vi "Create JSON Schema (Interactive).vi"(8 "error in (no error)":errorcluster, 9 "LV Object":variant, 11 "JSON Schema in":string) -> (0 "error out":errorcluster, 3 "JSON Schema out":string)   [LabVIEW 2019, in "JSON-Schema.lvlib"]
doc: "Interactively generates a JSON Schema for <b>LV object</b>, add additional, user-defined metadata, and merges with any <b>JSON Schema in</b>."
uses:
  <vilib>/JDP Science/JSONtext/Next JSON Value.vi
  <vilib>/JDP Science/JSONtext/String Subset.vi
  <vilib>/JDP Science/JSONtext/Parsing/Advance past next JSON Value (inlined COPY).vi
  <vilib>/JDP Science/JSONtext/Parsing/Advance past whitespace.vi
  <vilib>/JDP Science/JSONtext/Parsing/Advance past String.vi
  <vilib>/JDP Science/JSONtext/Parsing/Advance past Number.vi
  <vilib>/JDP Science/JSONtext/Parsing/Advance past Line Ending.vi
  <vilib>/JDP Science/JSONtext/Parsing/Parse Full Path or Item Name.vi
  <vilib>/JDP Science/JSONtext/Parsing/Advance past Array.vi
  <vilib>/JDP Science/JSONtext/Parsing/Advance past Object.vi
  <vilib>/JDP Science/JSONtext/support/Error Cluster From Code.vi
  <vilib>/JDP Science/JSONtext/Offset/Find Item Locations by Path.vi
  JSON-Schema.lvlib
  <vilib>/JDP Science/JSONtext/JSONtext.lvlib
  <vilib>/Utility/Data Type/NI_Data Type.lvlib
panel:
  in  "Write":bool
  in  "Table":bool
  in  "Load":bool
  in  "Path":path
  in  "Description":string
  in  "Title":string
  in  "Table":string[][](table)
  # "- This program will take a LV object and convert to a JSON Schema.\n   - If you don't wire anything to the LV Object terminal you can Load Object by Path.\n- After the initial JSON Schema is created, the Table will be filled with the relevant information.\n- Please update as appropriate and click Add Table to Schema.\n- Note: running Load Object will clear the previously loaded object and table."
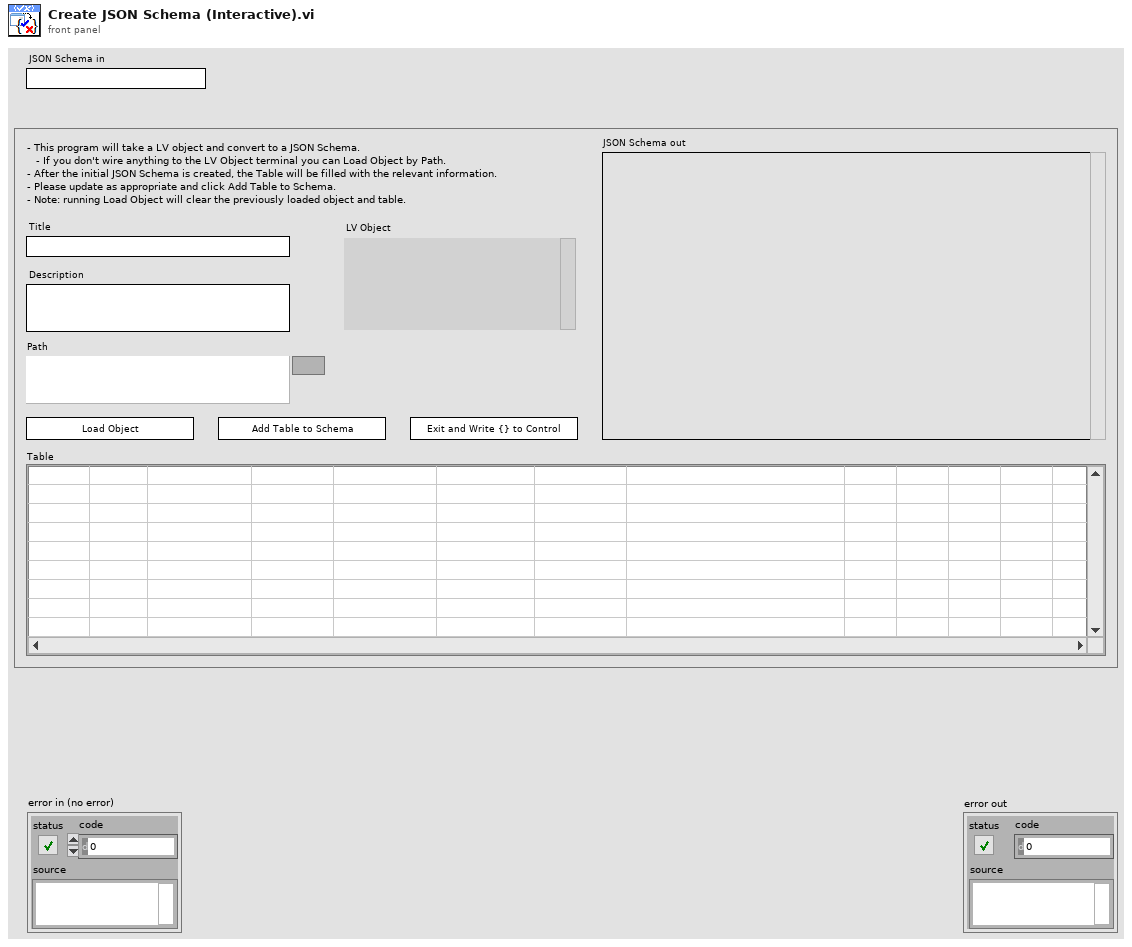
[diagram p1: front panel]
types:
  T1 = enum32{"Invalid", "Standard", "Closed", "Hidden", "Minimized", "Maximized"}
  T2 = enum32{"invalid app kind", "Development System", "Run Time System", "Student Edition", "Embedded LabVIEW", "Evaluation", "Custom"}
  T3 = cluster{"Core":cluster{"Current VI Reference":refnum<vi>, "Close Panel on Exit?":bool}, "JSON Schema":string, "LV Object":variant}
  T4 = cluster{"Current VI Reference":refnum<vi>, "Close Panel on Exit?":bool}
  T5 = typedef "JSONtext.lvlib/JSON Value Type.ctl" = enum16{"Not a JSON Value", "JSON Object", "JSON Array", "String", "Number", "true", "false", "null"}
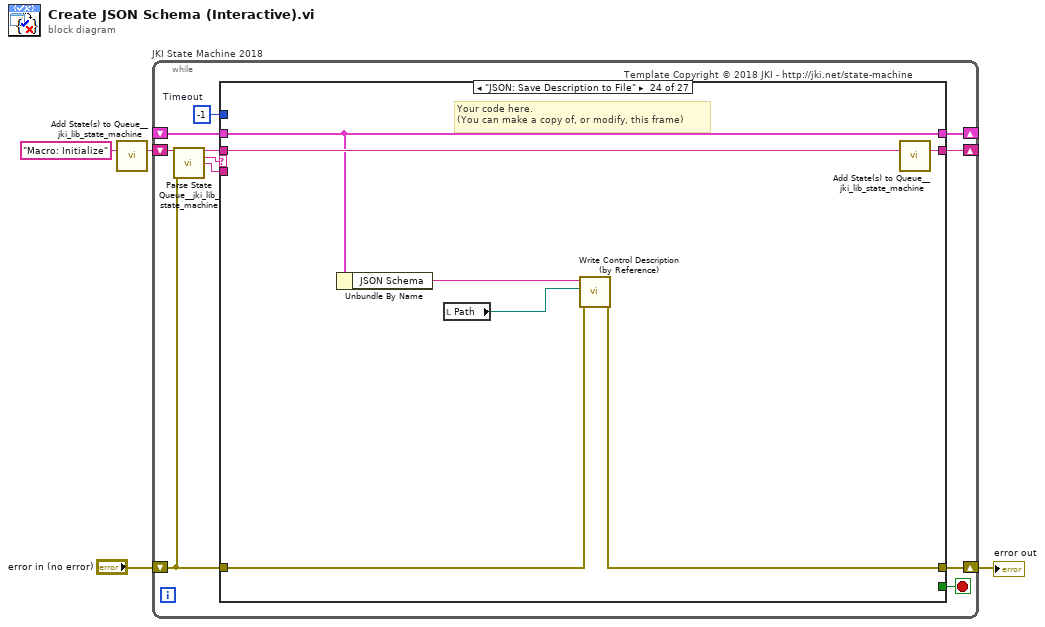
[diagram p0: block diagram]
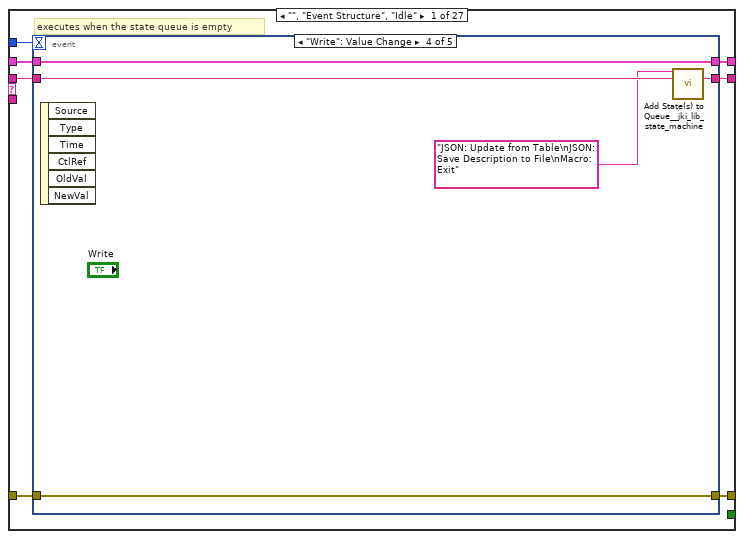
[diagram p2: hidden frame]
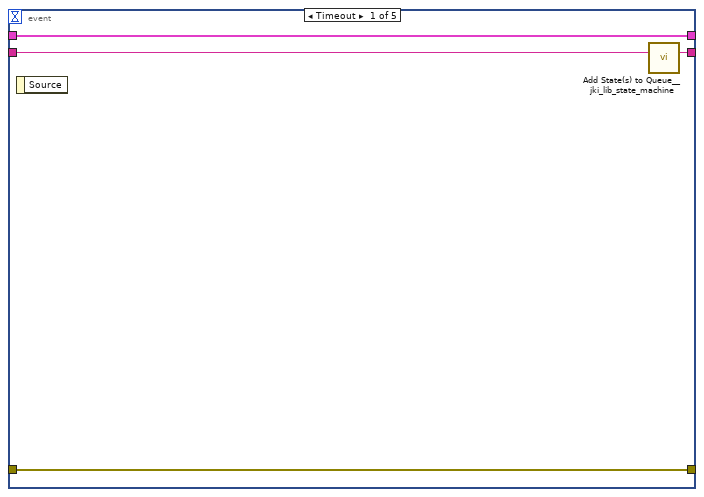
[diagram p3: hidden frame]
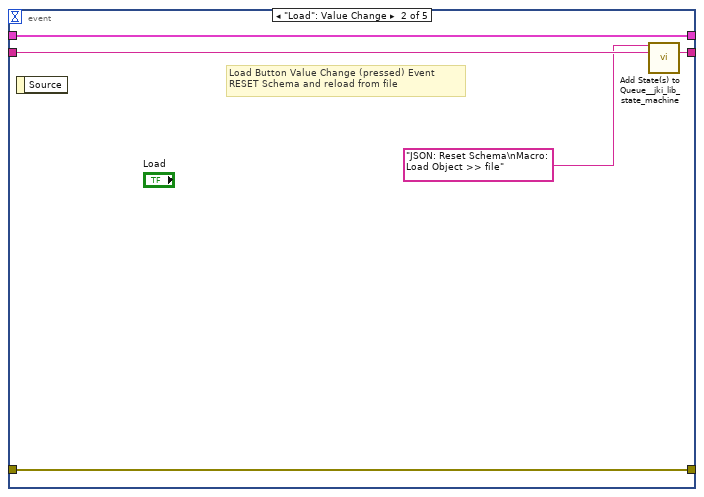
[diagram p4: hidden frame]
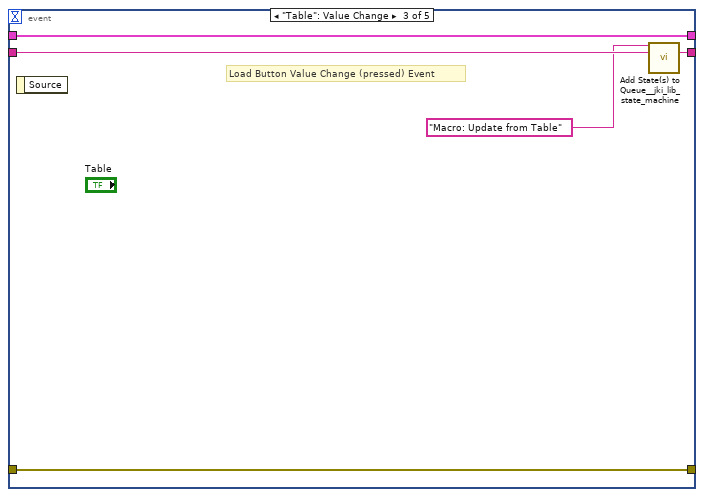
[diagram p5: hidden frame]
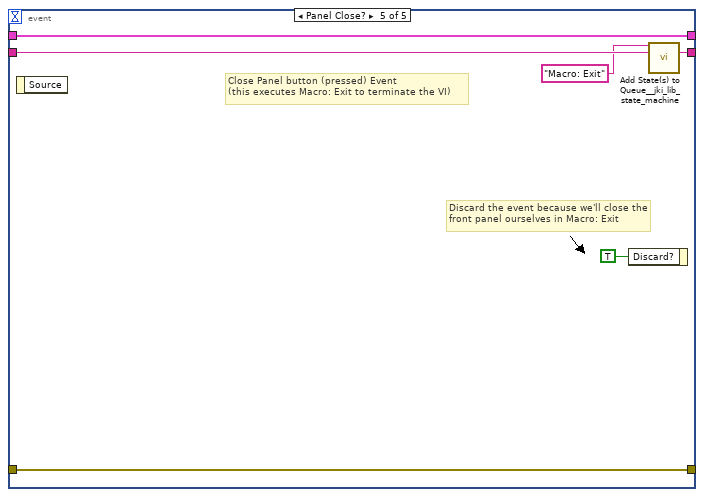
[diagram p6: hidden frame]
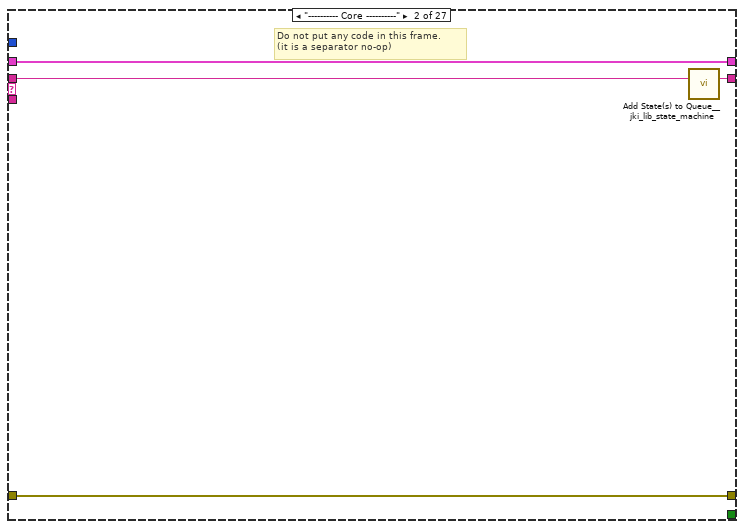
[diagram p7: hidden frame]
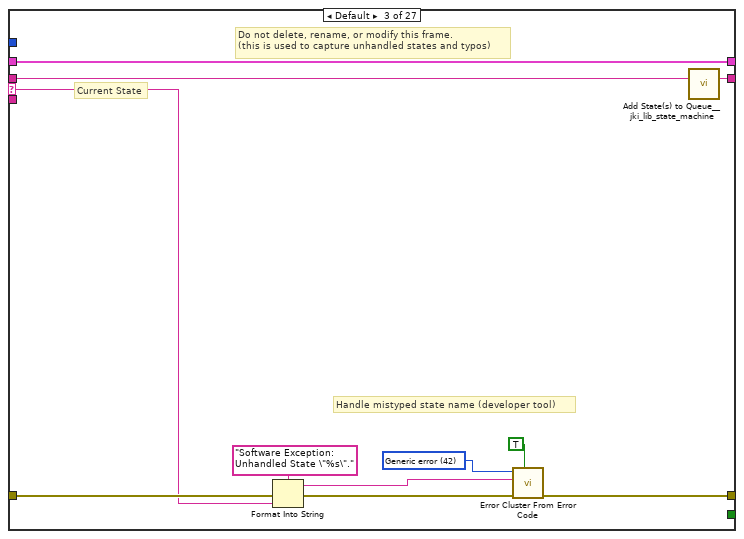
[diagram p8: hidden frame]
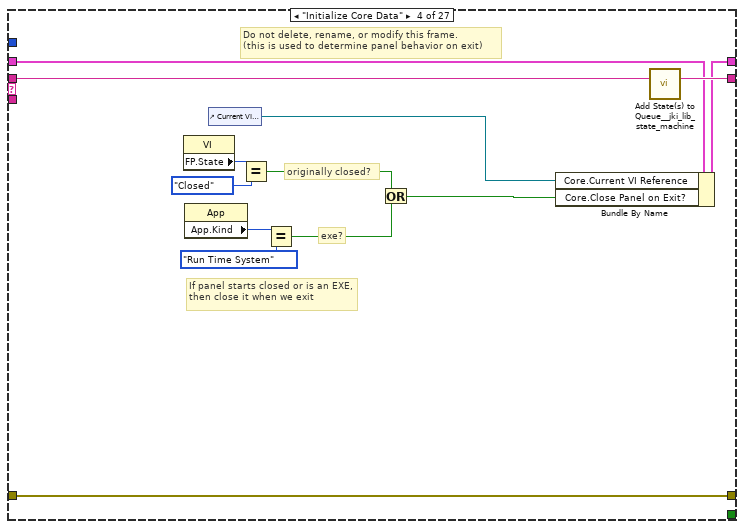
[diagram p9: hidden frame]
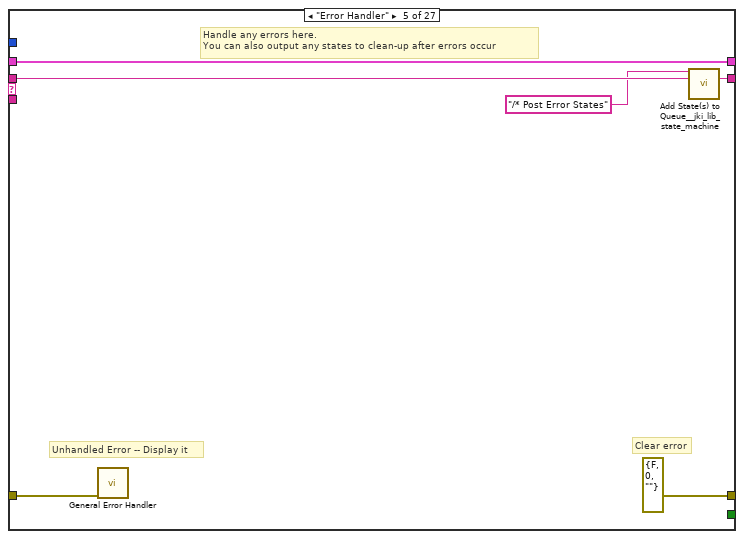
[diagram p10: hidden frame]
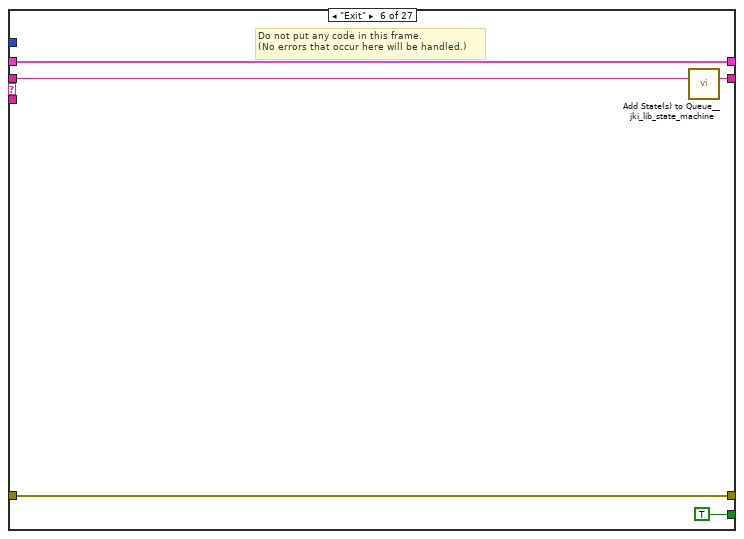
[diagram p11: hidden frame]
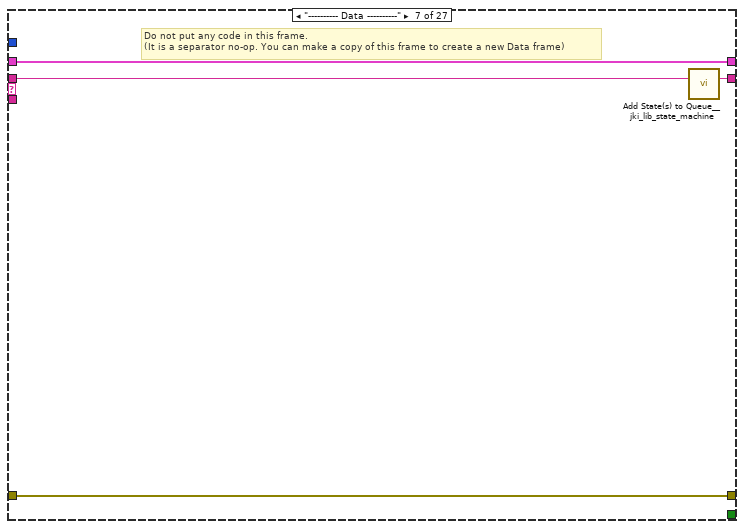
[diagram p12: hidden frame]
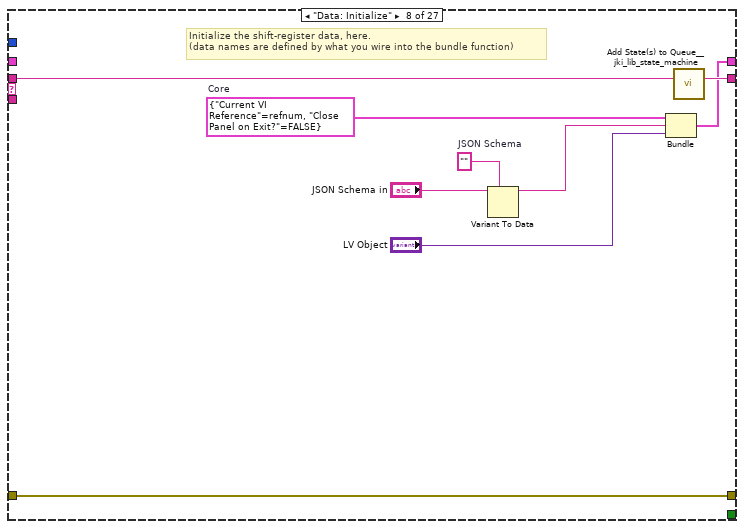
[diagram p13: hidden frame]
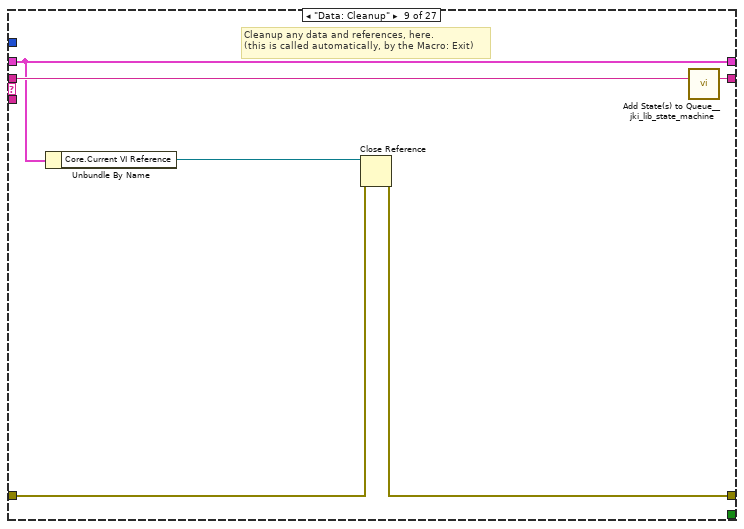
[diagram p14: hidden frame]
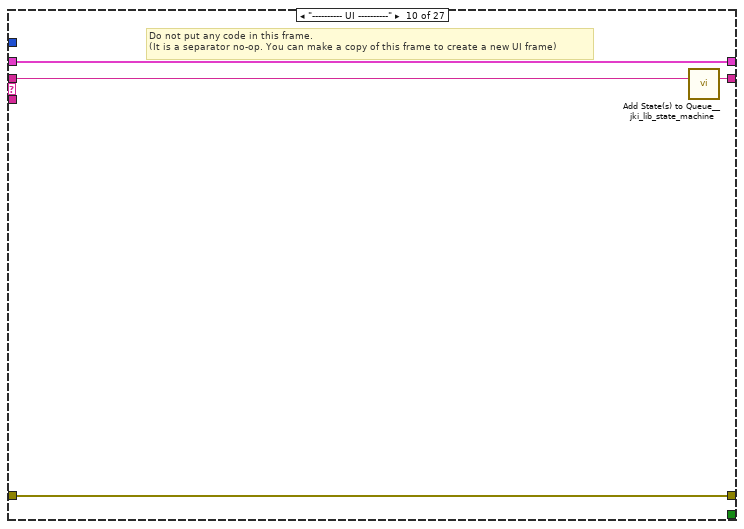
[diagram p15: hidden frame]
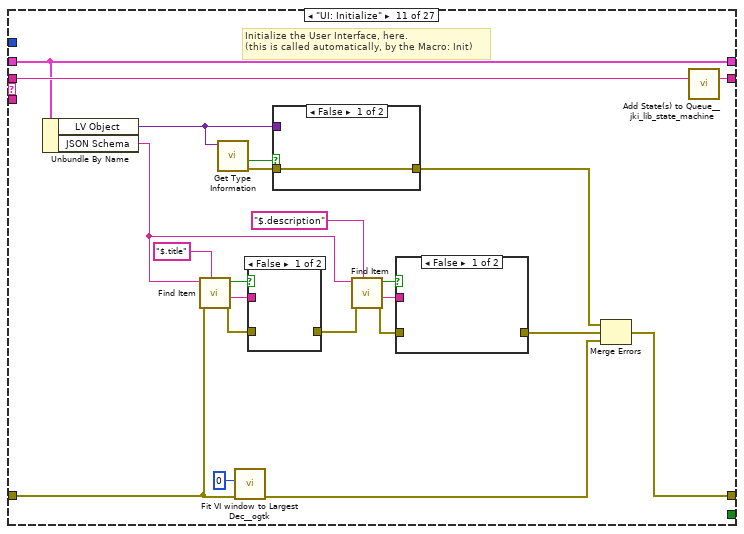
[diagram p16: hidden frame]
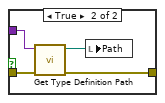
[diagram p17: hidden frame]
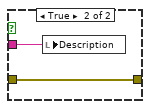
[diagram p18: hidden frame]
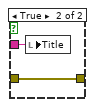
[diagram p19: hidden frame]
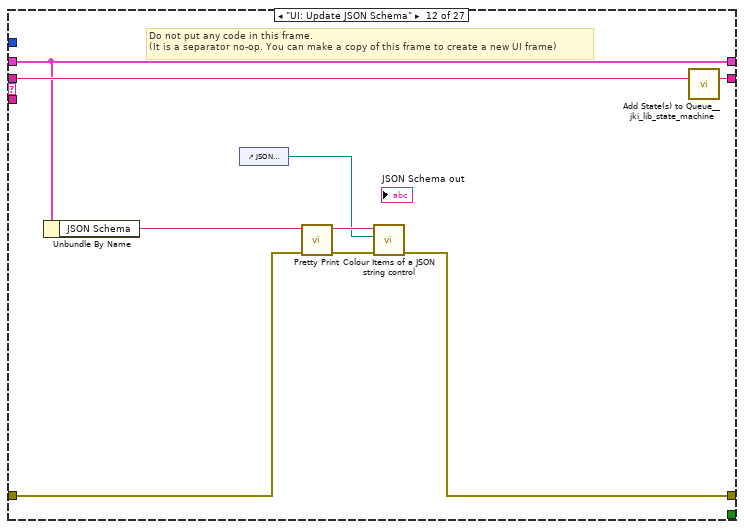
[diagram p20: hidden frame]
diagram:
  n1 = call <vilib>:"Add State(s) to Queue__jki_lib_state_machine.vi"("State(s) in (\"\")"="Macro: Initialize") -> ("States Out"=w4:string)  [unwired: 14 in]
  n2 = while "JKI State Machine 2018" {
    shift-right: [w8] -> _
    shift-left: _ -> [w7]
    shift-right: [w11] -> w1
    shift-left: "error in (no error)" -> [w5]
    shift-right: [w10] -> _
    shift-left: w4 -> [w12]
    stop <- w9 stop-if-true
    w6 = -1  # Timeout
    # "Template Copyright © 2018 JKI - http://jki.net/state-machine"
    n3 = call <vilib>:"Parse State Queue__jki_lib_state_machine.vi"("State Queue"=w12, "Error In (no error)"=w5) -> ("Remaining States"=w14:string, "Current State"=w15:string, "Arguments"=w13:string)  [unwired: 11 in]
    n4 = case shown="\"JSON: Save Description to File\"" w15 {
      selector: w15 -> [_ _ w52 _ _ _ _ _ _ _ _ _ _ _ _ _ _ _ _ _ _ _ _ _ _ _ _]
      tunnel: w14 -> [w22 w51 w56 w75 w81 w86 w90 w99 w105 w109 w131 w149 w155 w166 w235 w240 w252 w257 w267 w271 w281 w291 w303 w312 w321 w328 w337]
      tunnel: w13 -> [_ _ _ _ _ _ _ _ _ _ _ _ w150 w160 _ _ w248 _ _ _ _ _ _ _ _ _ _]
      tunnel: w7 -> [w20 w48 w54 w68 w78 w84 w87 _ w100 w106 w129 w146 w153 w162 w232 w237 w249 w254 w264 w268 w275 w285 w298 w308 w315 w325 w330]
      tunnel: [w19 w49 w58 w72 errorcluster {"status"=FALSE, "code"=0, "source"=""} ("error out") w83 w88 w94 w101 w107 w115 w142 w151 w163 w233 w238 w250 w255 w265 w269 w279 w289 w301 w310 w318 w323 w334] -> w11
      tunnel: w5 -> [w18 w49 w57 w72 w77 w83 w88 w94 w102 w107 w119 w141 w152 w164 w233 w238 w250 w255 w265 w269 w278 w288 w300 w309 w317 w322 w333]
      tunnel: [w21 w50 w55 w74 w80 w85 w89 w98 w104 w108 w130 w148 w154 w165 w234 w239 w251 w256 w266 w270 w280 w290 w302 w311 w320 w327 w336] -> w10
      tunnel: [_ _ _ _ _ TRUE _ _ _ _ _ _ _ _ _ _ _ _ _ _ _ _ _ _ _ _ _] -> w9
      tunnel: [w17 w48 w54 w73 w78 w84 w87 w97 w100 w106 w129 w146 w153 w162 w232 w237 w249 w254 w264 w268 w276 w286 w299 w308 w316 w325 w331] -> w8
      tunnel: w6 -> [w16 _ _ _ _ _ _ _ _ _ _ _ _ _ _ _ _ _ _ _ _ _ _ _ _ _ _]
      frame "", "Event Structure", "Idle" {
        # "executes when the state queue is empty"
        n5 = event shown="[3] \"Write\": Value Change" {
          selector: _ -> [_ _ _ _ _]
          dyn-events: _ -> [_ _ _ _ _]
          timeout: w16 -> [_ _ _ _ _]
          tunnel: w22 -> [w26 w31 w36 w41 w47]
          tunnel: [w25 w30 w35 w40 w46] -> w21
          tunnel: w20 -> [w23 w28 w33 w38 w44]
          tunnel: [w24 w29 w34 w39 w45] -> w19
          tunnel: w18 -> [w24 w29 w34 w39 w45]
          tunnel: [w23 w28 w33 w38 w44] -> w17
          event Timeout {
            n6 = event-data() -> ()  [unwired: 1 in, 1 out]
            n7 = call <vilib>:"Add State(s) to Queue__jki_lib_state_machine.vi"("State(s) in (\"\")"=w26) -> ("States Out"=w25:string)  [unwired: 14 in]
          }
          event "Load": Value Change {
            # "Load Button Value Change (pressed) Event\nRESET Schema and reload from file"
            n8 = event-data() -> ()  [unwired: 1 in, 1 out]
            n9 = call <vilib>:"Add State(s) to Queue__jki_lib_state_machine.vi"("State(s) in Front (\"\")"="JSON: Reset Schema\nMacro: Load Object >> file", "State(s) in (\"\")"=w31) -> ("States Out"=w30:string)  [unwired: 13 in]
          }
          event "Table": Value Change {
            # "Load Button Value Change (pressed) Event"
            n10 = event-data() -> ()  [unwired: 1 in, 1 out]
            n11 = call <vilib>:"Add State(s) to Queue__jki_lib_state_machine.vi"("State(s) in Front (\"\")"="Macro: Update from Table", "State(s) in (\"\")"=w36) -> ("States Out"=w35:string)  [unwired: 13 in]
          }
          event "Write": Value Change {
            n12 = event-data() -> ()  [unwired: 1 in, 6 out]
            n13 = call <vilib>:"Add State(s) to Queue__jki_lib_state_machine.vi"("State(s) in Front (\"\")"="JSON: Update from Table\nJSON: Save Description to File\nMacro: Exit", "State(s) in (\"\")"=w41) -> ("States Out"=w40:string)  [unwired: 13 in]
          }
          event Panel Close? {
            # "Discard the event because we'll close the front panel ourselves in Macro: Exit"
            # "Close Panel button (pressed) Event\n(this executes Macro: Exit to terminate the VI)"
            n14 = event-data() -> ()  [unwired: 1 in, 1 out]
            n15 = event-data("Discard?"=TRUE) -> ()  [unwired: 1 in, 1 out]
            n16 = call <vilib>:"Add State(s) to Queue__jki_lib_state_machine.vi"("State(s) in Front (\"\")"="Macro: Exit", "State(s) in (\"\")"=w47) -> ("States Out"=w46:string)  [unwired: 13 in]
          }
        }
      }
      frame "---------- Core ----------" {
        # "Do not put any code in this frame.\n(it is a separator no-op)"
        n17 = call <vilib>:"Add State(s) to Queue__jki_lib_state_machine.vi"("State(s) in (\"\")"=w51) -> ("States Out"=w50:string)  [unwired: 14 in]
      }
      frame Default {
        w61 = 42 items=["No error", "Argument error", "Memory is full", "Out of zone", "End of file", "File already open", "Generic file I/O error", "File not found", "File permission error", "Disk is full", "Duplicate path", "Too many files open", "System feature not enabled", "Resource file not found", "Cannot add resource", "Resource not found", "Image not found", "Image memory error", "Pen does not exist", "Config type invalid", "Config token not found", "Config parse error", "Config memory error", "Bad external code format", "Bad external code offset", "External code not present", "Null window", "Destroy window error", "Null menu", "Print aborted", "Bad print record", "Print driver error", "Windows error during printing", "Memory error during printing", "Print dialog error", "Generic print error", "Invalid device refnum", "Device not found", "Device parameter error", "Device unit error", "Cannot open device", "Device call aborted", "Generic error", "Cancelled by user", "Object ID too low", "Object ID too high", "Object not in heap", "Unknown heap", "Unknown object (invalid DefProc)", "Unknown object (DefProc not in table)", "Message out of range", "Invalid (null) method", "Unknown message", "Manager call not supported", "Bad address", "Network operation in progress", "Network operation timed out", "Connection is busy", "Network attribute not supported", "Network error", "Address in use", "System out of memory", "Connection aborted", "Connection refused", "Not connected", "Already connected", "Connection closed", "Initialization error (interapplication manager)", "Bad occurrence", "Wait on unbound occurrence handler", "Occurrence queue overflow", "Datalog type conflict", "Unused", "Unrecognized type (interapplication manager)", "Memory corrupt", "Failed to make temporary DLL", "Old CIN version", "Drag socket not found", "Failed to load drop-object", "Failed to register OLE object", "Failed to release OLE object", "Format specifier type mismatch", "Unknown format specifier", "Too few format specifiers", "Too many format specifiers", "Scan failed", "Newer CIN version", "Error converting to variant", "Runtime menu error", "Password tampered", "Variant attribute not found", "Incompatible variant data type", "Event data is not available", "Event Store is not present", "Occurrence is not found", "Event Queue is not created", "Event info is not available", "Refnum passed is NULL", "Error retrieving Class GUID", "Error retrieving CoClass GUID", "Error retrieving TypeLib GUID.", "Bad built application magic bytes.", "Specific driver is different from the specific driver associated with the Logical Name.", "There is no session opened to the class driver.", "Max Error", "MAX - Error with config objects", "MAX - Error loading configuration", "MAX - Group not supported"]
        # "Current State"
        # "Do not delete, rename, or modify this frame.\n(this is used to capture unhandled states and typos)"
        # "Handle mistyped state name (developer tool)"
        n18 = Format Into String(format string="Software Exception: Unhandled State \"%s\"." ("message"), error in=w57, w52) -> (resulting string=w60:string, error out=w59:errorcluster)  [unwired: 1 in]
        n19 = call <vilib>:"Error Cluster From Error Code.vi"("show call chain? (False)"=TRUE, "error in (no error)"=w59, "error message (\"\")"=w60, "error code (0)"=w61) -> ("error out"=w58:errorcluster)  [unwired: 5 in]
        n20 = call <vilib>:"Add State(s) to Queue__jki_lib_state_machine.vi"("State(s) in (\"\")"=w56) -> ("States Out"=w55:string)  [unwired: 14 in]
      }
      frame "Initialize Core Data" {
        # "Do not delete, rename, or modify this frame.\n(this is used to determine panel behavior on exit)"
        # "originally closed?"
        # "exe?"
        # "If panel starts closed or is an EXE, then close it when we exit"
        n21 = property class="VI"() -> ("FP.State"=w65:T1)  [unwired: 2 in, 2 out]
        n22 = property class="App"() -> ("App.Kind"=w71:T2)  [unwired: 2 in, 2 out]
        n23 = control-ref of="Current VI Reference"() -> (w66:refnum<vi>)
        n24 = Equal?(x=w65, y=T1."Closed" ("Front Panel Window:State")) -> (x = y?=w63:bool)
        n25 = Equal?(x=w71, y=T2."Run Time System" ("Application:Kind")) -> (x = y?=w69:bool)
        n26 = Or(x=w63, y=w69) -> (x .or. y?=w67:bool)
        n27 = Bundle By Name(cluster=w68, "Core.Current VI Reference"=w66, "Core.Close Panel on Exit?"=w67) -> (w73:T3)
        n28 = call <vilib>:"Add State(s) to Queue__jki_lib_state_machine.vi"("State(s) in (\"\")"=w75) -> ("States Out"=w74:string)  [unwired: 14 in]
      }
      frame "Error Handler" {
        # "Unhandled Error -- Display it"
        # "Handle any errors here.\nYou can also output any states to clean-up after errors occur"
        # "Clear error"
        n29 = call <vilib>:"General Error Handler.vi"("error in (no error)"=w77) -> ()  [unwired: 10 in, 5 out]
        n30 = call <vilib>:"Add State(s) to Queue__jki_lib_state_machine.vi"("State(s) in Front (\"\")"="/* Post Error States", "State(s) in (\"\")"=w81) -> ("States Out"=w80:string)  [unwired: 13 in]
      }
      frame "Exit" {
        # "Do not put any code in this frame.\n(No errors that occur here will be handled.)"
        n31 = call <vilib>:"Add State(s) to Queue__jki_lib_state_machine.vi"("State(s) in (\"\")"=w86) -> ("States Out"=w85:string)  [unwired: 14 in]
      }
      frame "---------- Data ----------" {
        # "Do not put any code in this frame.\n(It is a separator no-op. You can make a copy of this frame to create a new Data frame)"
        n32 = call <vilib>:"Add State(s) to Queue__jki_lib_state_machine.vi"("State(s) in (\"\")"=w90) -> ("States Out"=w89:string)  [unwired: 14 in]
      }
      frame "Data: Initialize" {
        w93 = ""  # JSON Schema
        w96 = T4 {"Current VI Reference"=refnum, "Close Panel on Exit?"=FALSE}  # Core
        # "Initialize the shift-register data, here.\n(data names are defined by what you wire into the bundle function)"
        n33 = Variant To Data(type=w93, Variant="JSON Schema in") -> (data=w92:string)  [unwired: 1 in, 1 out]
        n34 = Bundle("Core"=w96, "JSON Schema"=w92, "LV Object"="LV Object") -> (w97:T3)  [unwired: 1 in]
        n35 = call <vilib>:"Add State(s) to Queue__jki_lib_state_machine.vi"("State(s) in (\"\")"=w99) -> ("States Out"=w98:string)  [unwired: 14 in]
      }
      frame "Data: Cleanup" {
        # "Cleanup any data and references, here.\n(this is called automatically, by the Macro: Exit)"
        n36 = Unbundle By Name(w100) -> ("Core.Current VI Reference"=w103:refnum<vi>)
        n37 = Close Reference(reference=w103, error in (no error)=w102) -> (error out=w101:errorcluster)
        n38 = call <vilib>:"Add State(s) to Queue__jki_lib_state_machine.vi"("State(s) in (\"\")"=w105) -> ("States Out"=w104:string)  [unwired: 14 in]
      }
      frame "---------- UI ----------" {
        # "Do not put any code in this frame.\n(It is a separator no-op. You can make a copy of this frame to create a new UI frame)"
        n39 = call <vilib>:"Add State(s) to Queue__jki_lib_state_machine.vi"("State(s) in (\"\")"=w109) -> ("States Out"=w108:string)  [unwired: 14 in]
      }
      frame "UI: Initialize" {
        # "Initialize the User Interface, here.\n(this is called automatically, by the Macro: Init)"
        n40 = Unbundle By Name(w129) -> ("LV Object"=w112:variant, "JSON Schema"=w111:string)
        n41 = call <vilib>:"Find Item.vi"("$Path or Item Name"="$.title", "error in (no error)"=w119, "JSON"=w111) -> ("error out"=w124:errorcluster, "<JSON>"=w127:string, "Found"=w125:bool)  [unwired: 5 in, 1 out]
        n42 = call <vilib>:"Get Type Information.vi"("variant"=w112) -> ("error out"=w117:errorcluster, "type definition"=w118:bool)  [unwired: 6 in, 3 out]
        n43 = call <userlib>:"Fit VI window to Largest Dec__ogtk.vi"("error in (no error)"=w119, "border spacing (2 px)"=0) -> ("error out"=w113:errorcluster)  [unwired: 4 in, 1 out]
        n44 = case shown="False" w125 {
          tunnel: w127 -> [_ w140]
          tunnel: w124 -> [_ w139]
          tunnel: [_ w139] -> w123
          frame False {
          }
          frame True {
            n45 = local write "Title"(w140) -> ()
          }
        }
        n46 = case shown="False" w118 {
          tunnel: w112 -> [_ w136]
          tunnel: w117 -> [w132 w134]
          tunnel: [w132 w133] -> w116
          frame False {
          }
          frame True {
            n47 = call <vilib>:"Get Type Definition Path.vi"("error in (no error)"=w134, "variant"=w136) -> ("error out"=w133:errorcluster, "type definition path"=w135:path)  [unwired: 8 in]
            n48 = local write "Path"(w135) -> ()
          }
        }
        n49 = call <vilib>:"Find Item.vi"("$Path or Item Name"="$.description", "error in (no error)"=w123, "JSON"=w111) -> ("error out"=w120:errorcluster, "<JSON>"=w121:string, "Found"=w122:bool)  [unwired: 5 in, 1 out]
        n50 = case shown="False" w122 {
          tunnel: w121 -> [_ w138]
          tunnel: [_ w137] -> w114
          tunnel: w120 -> [_ w137]
          frame False {
          }
          frame True {
            n51 = local write "Description"(w138) -> ()
          }
        }
        n52 = Merge Errors(w116, w114, w113) -> (w115:errorcluster)
        n53 = call <vilib>:"Add State(s) to Queue__jki_lib_state_machine.vi"("State(s) in (\"\")"=w131) -> ("States Out"=w130:string)  [unwired: 14 in]
      }
      frame "UI: Update JSON Schema" {
        # "Do not put any code in this frame.\n(It is a separator no-op. You can make a copy of this frame to create a new UI frame)"
        n54 = Unbundle By Name(w146) -> ("JSON Schema"=w145:string)
        n55 = control-ref of="JSON Schema out"() -> (w144:refnum<vi>)
        n56 = call <vilib>:"Pretty Print.vi"("error in (no error)"=w141, "JSON"=w145) -> ("error out"=w143:errorcluster, "<JSON>"=w147:string)  [unwired: 7 in, 1 out]
        n57 = call <vilib>:"Colour Items of a JSON string control.vi"("error in (no error)"=w143, "String Control"=w144, "JSON"=w147) -> ("error out"=w142:errorcluster)  [unwired: 8 in]
        n58 = call <vilib>:"Add State(s) to Queue__jki_lib_state_machine.vi"("State(s) in (\"\")"=w149) -> ("States Out"=w148:string)  [unwired: 14 in]
      }
      frame "UI: Cursor Set" {
        # "Argument"
        # "Set and Unset Cursor Busy.\n(Usage: \"UI: Cursor Set >> Busy|Idle\")"
        n59 = case shown="\"Idle\", Default" w150 {
          tunnel: w152 -> [w157 w159]
          tunnel: [w156 w158] -> w151
          frame "Idle", Default {
            n60 = call <vilib>:"Unset Busy.vi"("error in (no error)"=w157) -> ("error out"=w156:errorcluster)  [unwired: 10 in]
          }
          frame "Busy" {
            n61 = call <vilib>:"Set Busy.vi"("error in (no error)"=w159) -> ("error out"=w158:errorcluster)  [unwired: 9 in, 1 out]
          }
        }
        n62 = call <vilib>:"Add State(s) to Queue__jki_lib_state_machine.vi"("State(s) in (\"\")"=w155) -> ("States Out"=w154:string)  [unwired: 14 in]
      }
      frame "UI: Front Panel State" {
        # "Argument"
        # "Set Front Panel Open or Closed\n(Usage: \"UI: Front Panel State >> Open|Close\")"
        n63 = Unbundle By Name(w162) -> ("Core.Current VI Reference"=w161:refnum<vi>)
        n64 = case shown="\"Open\", \"Standard\", Default" w160 {
          tunnel: w164 -> [w172 w187 w198 w211 w224]
          tunnel: [w174 w188 w200 w213 w226] -> w163
          tunnel: w161 -> [w173 w185 w199 w212 w225]
          frame "Open", "Standard", Default {
            w167 = T1."Standard" ("State")
            n65 = property class="VI"(reference=w173, error in=w172) -> (reference out=w170:refnum<vi>, error out=w171:errorcluster, "FP.State"=w169:T1)
            n66 = Not Equal?(x=w169, y=w167) -> (x != y?=w168:bool)
            n67 = case shown="False" w168 {
              tunnel: [w178 w180] -> w174
              tunnel: w171 -> [w177 w180]
              tunnel: w170 -> [w176 _]
              tunnel: w167 -> [w175 _]
              frame True {
                n68 = invoke class="VI" method="FP.Open"(reference=w176, error in=w177, "Activate"=TRUE, "State"=w175) -> (error out=w178:errorcluster)  [unwired: 1 in, 4 out]
              }
              frame False {
              }
            }
          }
          frame "Close", "Closed" {
            n69 = property class="VI"(reference=w185, error in=w187) -> (reference out=w184:refnum<vi>, error out=w186:errorcluster, "FP.State"=w182:T1)
            n70 = Not Equal?(x=w182, y=T1."Closed" ("Front Panel Window:State")) -> (x != y?=w181:bool)
            n71 = case shown="True" w181 {
              tunnel: [w189 w192] -> w188
              tunnel: w186 -> [w189 w191]
              tunnel: w184 -> [_ w190]
              frame False {
              }
              frame True {
                n72 = invoke class="VI" method="FP.Close"(reference=w190, error in=w191) -> (error out=w192:errorcluster)  [unwired: 1 in, 2 out]
              }
            }
          }
          frame "Hidden", "Hide" {
            w193 = T1."Hidden" ("State")
            n73 = property class="VI"(reference=w199, error in=w198) -> (reference out=w196:refnum<vi>, error out=w197:errorcluster, "FP.State"=w195:T1)
            n74 = Not Equal?(x=w195, y=w193) -> (x != y?=w194:bool)
            n75 = case shown="True" w194 {
              tunnel: [w204 w205] -> w200
              tunnel: w197 -> [w203 w205]
              tunnel: w196 -> [w202 _]
              tunnel: w193 -> [w201 _]
              frame True {
                n76 = invoke class="VI" method="FP.Open"(reference=w202, error in=w203, "State"=w201) -> (error out=w204:errorcluster)  [unwired: 2 in, 4 out]
              }
              frame False {
              }
            }
          }
          frame "Minimize", "Minimized" {
            w206 = T1."Minimized" ("State")
            n77 = property class="VI"(reference=w212, error in=w211) -> (reference out=w209:refnum<vi>, error out=w210:errorcluster, "FP.State"=w208:T1)
            n78 = Not Equal?(x=w208, y=w206) -> (x != y?=w207:bool)
            n79 = case shown="True" w207 {
              tunnel: [w217 w218] -> w213
              tunnel: w210 -> [w216 w218]
              tunnel: w209 -> [w215 _]
              tunnel: w206 -> [w214 _]
              frame True {
                n80 = invoke class="VI" method="FP.Open"(reference=w215, error in=w216, "State"=w214) -> (error out=w217:errorcluster)  [unwired: 2 in, 4 out]
              }
              frame False {
              }
            }
          }
          frame "Maximize", "Maximized" {
            w219 = T1."Maximized" ("State")
            n81 = property class="VI"(reference=w225, error in=w224) -> (reference out=w222:refnum<vi>, error out=w223:errorcluster, "FP.State"=w221:T1)
            n82 = Not Equal?(x=w221, y=w219) -> (x != y?=w220:bool)
            n83 = case shown="True" w220 {
              tunnel: [w230 w231] -> w226
              tunnel: w223 -> [w229 w231]
              tunnel: w222 -> [w228 _]
              tunnel: w219 -> [w227 _]
              frame True {
                n84 = invoke class="VI" method="FP.Open"(reference=w228, error in=w229, "State"=w227) -> (error out=w230:errorcluster)  [unwired: 2 in, 4 out]
              }
              frame False {
              }
            }
          }
        }
        n85 = call <vilib>:"Add State(s) to Queue__jki_lib_state_machine.vi"("State(s) in (\"\")"=w166) -> ("States Out"=w165:string)  [unwired: 14 in]
      }
      frame "---------- Macro ----------" {
        # "Do not put any code in this frame.\n(It is a separator no-op. You can make a copy of this frame to create a new Macro frame)"
        n86 = call <vilib>:"Add State(s) to Queue__jki_lib_state_machine.vi"("State(s) in (\"\")"=w235) -> ("States Out"=w234:string)  [unwired: 14 in]
      }
      frame "Macro: Initialize" {
        # "Initialization Macro\n(This is called once, when the VI starts)"
        n87 = call <vilib>:"Add State(s) to Queue__jki_lib_state_machine.vi"("State(s) in Front (\"\")"="Data: Initialize\nInitialize Core Data\nUI: Initialize\nUI: Front Panel State >> Open\nMacro: Load Object", "State(s) in (\"\")"=w240) -> ("States Out"=w239:string)  [unwired: 13 in]
      }
      frame "Macro: Load Object" {
        # "Do not put any code in this frame.\n(It is a separator no-op. You can make a copy of this frame to create a new Macro frame)"
        n88 = Equal?(x=w248, y="file") -> (x = y?=w246:bool)
        n89 = Select(t="", s=w246, f="//") -> (s? t:f=w242:string)
        n90 = Format Into String(format string="JSON: Initialize Schema\n%sJSON: Load Object from File\nJSON: Process Object\nJSON: Create Table\nUI: Update JSON Schema" ("State(s) in Front (\"\")"), w242) -> (resulting string=w244:string)  [unwired: 2 in, 1 out]
        n91 = call <vilib>:"Add State(s) to Queue__jki_lib_state_machine.vi"("State(s) in Front (\"\")"=w244, "State(s) in (\"\")"=w252) -> ("States Out"=w251:string)  [unwired: 13 in]
      }
      frame "Macro: Update from Table" {
        # "Do not put any code in this frame.\n(It is a separator no-op. You can make a copy of this frame to create a new Macro frame)"
        n92 = call <vilib>:"Add State(s) to Queue__jki_lib_state_machine.vi"("State(s) in Front (\"\")"="JSON: Update from Table\nUI: Update JSON Schema" ("State(s) in Front (\"\")"), "State(s) in (\"\")"=w257) -> ("States Out"=w256:string)  [unwired: 13 in]
      }
      frame "Macro: Exit" {
        # "Exit Macro\n(This is called once, when the VI exits)"
        n93 = Unbundle By Name(w264) -> ("Core.Close Panel on Exit?"=w263:bool)
        n94 = Select(t="UI: Front Panel State >> Close", s=w263, f="") -> (s? t:f=w260:string)
        n95 = call <vilib>:"Add State(s) to Queue__jki_lib_state_machine.vi"("State(s) in (\"\")"=w260, "State(s) at Back (\"\")"="Data: Cleanup\nExit") -> ("States Out"=w258:string)  [unwired: 13 in]
        n96 = call <vilib>:"Add State(s) to Queue__jki_lib_state_machine.vi"("State(s) in Front (\"\")"=w258, "State(s) in (\"\")"=w267) -> ("States Out"=w266:string)  [unwired: 13 in]
      }
      frame "---------- JSON ----------" {
        # "Template Separator\n(You can make a copy of, or modify, this frame)"
        n97 = call <vilib>:"Add State(s) to Queue__jki_lib_state_machine.vi"("State(s) in (\"\")"=w271) -> ("States Out"=w270:string)  [unwired: 14 in]
      }
      frame "JSON: Initialize Schema" {
        # "1. initialize JSON Schema"
        n98 = Unbundle By Name(w275) -> ("JSON Schema"=w274:string)
        n99 = call "Initialize JSON Schema.vi"("error in (no error)"=w278, "Description"="Description", "Title"="Title", "JSON Schema in"=w274) -> ("error out"=w279:errorcluster, "JSON Schema out"=w277:string)  [unwired: 6 in]
        n100 = Bundle By Name(cluster=w275, "JSON Schema"=w277) -> (w276:T3)
        n101 = call <vilib>:"Add State(s) to Queue__jki_lib_state_machine.vi"("State(s) in (\"\")"=w281) -> ("States Out"=w280:string)  [unwired: 14 in]
      }
      frame "JSON: Reset Schema" {
        # "1. initialize JSON Schema"
        n102 = local read "Description"() -> (w282:string)
        n103 = local read "Title"() -> (w284:string)
        n104 = call "Initialize JSON Schema.vi"("error in (no error)"=w288, "Description"=w282, "Title"=w284, "JSON Schema in"="{}") -> ("error out"=w289:errorcluster, "JSON Schema out"=w287:string)  [unwired: 6 in]
        n105 = Bundle By Name(cluster=w285, "JSON Schema"=w287) -> (w286:T3)
        n106 = call <vilib>:"Add State(s) to Queue__jki_lib_state_machine.vi"("State(s) in (\"\")"=w291) -> ("States Out"=w290:string)  [unwired: 14 in]
      }
      frame "JSON: Load Object from File" {
        # "Your code here.\n(You can make a copy of, or modify, this frame)"
        n107 = Unbundle By Name(w298) -> ("JSON Schema"=w293:string)
        n108 = call "Read Control Description (by Reference).vi"("error in (no error)"=w300, "ctl path"="Path") -> ("error out"=w301:errorcluster, "Value"=w292:variant, "VI Description"=w295:string)  [unwired: 7 in]
        n109 = call <vilib>:"JSON type.vi"("JSON"=w295) -> ("JSON Value Type"=w297:T5)  [unwired: 9 in, 1 out]
        n110 = case shown="Default" w297 {
          tunnel: [w304 w305] -> w296
          tunnel: w295 -> [_ w305]
          tunnel: w293 -> [w304 _]
          frame Default {
          }
          frame "JSON Object" {
          }
        }
        n111 = local write "LV Object"(w292) -> ()
        n112 = Bundle By Name(cluster=w298, "JSON Schema"=w296, "LV Object"=w292) -> (w299:T3)
        n113 = call <vilib>:"Add State(s) to Queue__jki_lib_state_machine.vi"("State(s) in (\"\")"=w303) -> ("States Out"=w302:string)  [unwired: 14 in]
      }
      frame "JSON: Save Description to File" {
        # "Your code here.\n(You can make a copy of, or modify, this frame)"
        n114 = Unbundle By Name(w308) -> ("JSON Schema"=w306:string)
        n115 = local read "Path"() -> (w307:path)
        n116 = call "Write Control Description (by Reference).vi"("error in (no error)"=w309, "ctl path"=w307, "VI Description in"=w306) -> ("error out"=w310:errorcluster)  [unwired: 7 in, 1 out]
        n117 = call <vilib>:"Add State(s) to Queue__jki_lib_state_machine.vi"("State(s) in (\"\")"=w312) -> ("States Out"=w311:string)  [unwired: 14 in]
      }
      frame "JSON: Process Object" {
        # "Template Separator\n(You can make a copy of, or modify, this frame)"
        n118 = Unbundle By Name(w315) -> ("JSON Schema"=w319:string, "LV Object"=w313:variant)
        n119 = call "Add Object to JSON Schema.vi"("error in (no error)"=w317, "Object"=w313, "JSON Schema in"=w319) -> ("error out"=w318:errorcluster, "JSON Schema out"=w314:string)  [unwired: 7 in]
        n120 = Bundle By Name(cluster=w315, "JSON Schema"=w314) -> (w316:T3)
        n121 = call <vilib>:"Add State(s) to Queue__jki_lib_state_machine.vi"("State(s) in (\"\")"=w321) -> ("States Out"=w320:string)  [unwired: 14 in]
      }
      frame "JSON: Create Table" {
        # "Template Separator\n(You can make a copy of, or modify, this frame)"
        n122 = Unbundle By Name(w325) -> ("JSON Schema"=w324:string)
        n123 = call "JSON Schema to Table.vi"("error in (no error)"=w322, "JSON Schema in"=w324) -> ("error out"=w323:errorcluster, "Table"=w326:string[][])  [unwired: 7 in, 1 out]
        n124 = local write "Table"(w326) -> ()
        n125 = call <vilib>:"Add State(s) to Queue__jki_lib_state_machine.vi"("State(s) in (\"\")"=w328) -> ("States Out"=w327:string)  [unwired: 14 in]
      }
      frame "JSON: Update from Table" {
        # "Template Separator\n(You can make a copy of, or modify, this frame)"
        n126 = Unbundle By Name(w330) -> ("JSON Schema"=w332:string)
        n127 = call "Table to JSON Schema.vi"("error in (no error)"=w333, "Table"="Table", "JSON Schema in"=w332) -> ("error out"=w334:errorcluster, "JSON Schema out"=w329:string)  [unwired: 7 in]
        n128 = Bundle By Name(cluster=w330, "JSON Schema"=w329) -> (w331:T3)
        n129 = call <vilib>:"Add State(s) to Queue__jki_lib_state_machine.vi"("State(s) in (\"\")"=w337) -> ("States Out"=w336:string)  [unwired: 14 in]
      }
    }
  }
  "error out" <- w1
